vi "Drone video to IMAQ - Main (SubVI).vi"() -> (0 "error out":errorcluster, 3 "raw image":T1)   [LabVIEW 2014]
uses:
  <vilib>/vision/Image Controls.llb/IMAQ Image.ctl
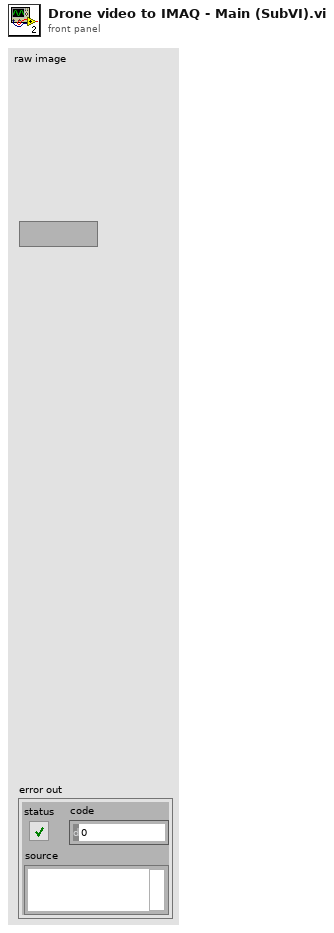
[diagram p1: front panel]
types:
  T1 = typedef "IMAQ Image.ctl" = refnum<image>
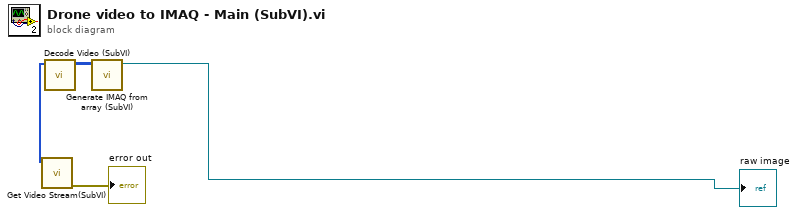
[diagram p0: block diagram]
diagram:
  n1 = call "Get Video Stream(SubVI).vi"() -> ("error out"=→"error out":errorcluster, "ImgData"=w1:u8[])  [unwired: 10 in]
  n2 = call "Decode Video (SubVI).vi"("ImgData"=w1) -> ("Array"=w2:u32[][])  [unwired: 9 in, 1 out]
  n3 = call "Generate IMAQ from array (SubVI).vi"("Array"=w2) -> ("Refnum out"=→"raw image":T1)  [unwired: 10 in]
